vi "Command_Turn_To_Heading.vi"(0 "Startup":bool, 2 "Heading":dbl, 3 "Timeout":dbl=3.0) -> (5 "Reinit":bool, 6 "Completed":bool=TRUE, 7 "Speeds":dbl[](array[numeric]))   [LabVIEW 2018]
uses:
  Global_Variables/Sensor_Values.vi
panel:
  in  "Kd":dbl=0.0012 format="%#_13g"
  in  "Ki":dbl=0.0001 format="%#_13g"
  in  "Kp":dbl=0.01 format="%#_13g"
  out "Waveform Chart":cluster{"Heading":dbl, "Yaw":dbl}(graph)
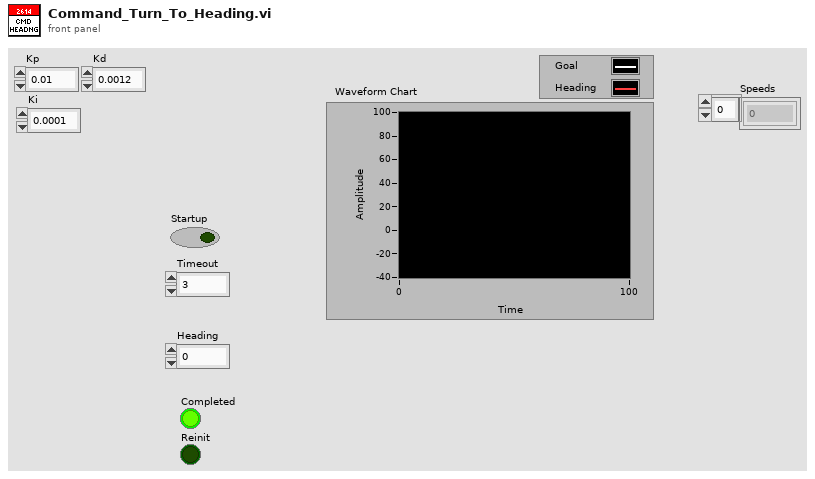
[diagram p1: front panel]
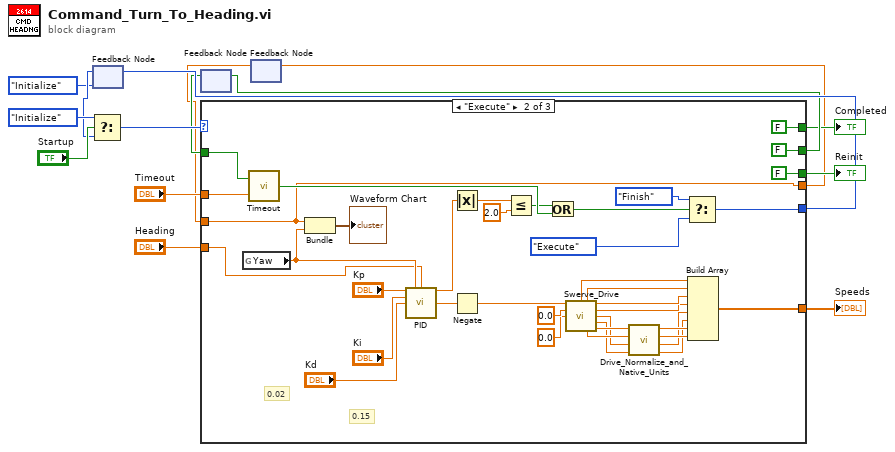
[diagram p0: block diagram]
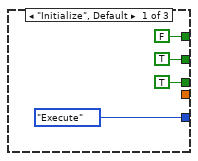
[diagram p2: hidden frame]
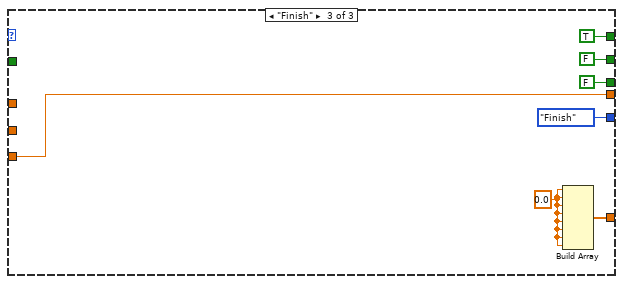
[diagram p3: hidden frame]
diagram:
  n1 = feedback #1(enum16{"Initialize", "Execute", "Finish"}."Initialize" ("f")) -> (w11:enum16{"Initialize", "Execute", "Finish"})
  n2 = Select(t=enum16{"Initialize", "Execute", "Finish"}."Initialize", s="Startup", f=w11) -> (s? t:f=w15:enum16{"Initialize", "Execute", "Finish"})
  n3 = feedback #2() -> (w9:bool)  [unwired: 1 in]
  n4 = feedback #3() -> (w1:dbl)  [unwired: 1 in]
  n5 = case shown="\"Execute\"" w15 {
    tunnel: [enum16{"Initialize", "Execute", "Finish"}."Execute" w54 enum16{"Initialize", "Execute", "Finish"}."Finish" ("f")] -> w12
    tunnel: w9 -> [_ w52 _]
    tunnel: [TRUE FALSE FALSE] -> w10
    tunnel: [FALSE FALSE TRUE] -> w8
    tunnel: [TRUE FALSE FALSE] -> w7
    tunnel: "Timeout" -> [_ w48 _]
    tunnel: "Heading" -> [_ w28 w58]
    tunnel: [_ w43 w60] -> w3
    tunnel: [_ w31 w58] -> w2
    tunnel: w1 -> [_ w31 _]
    frame "Initialize", Default {
    }
    frame "Execute" {
      # "0.02"
      # "0.15"
      n6 = global read "Sensor_Values.vi" "Yaw"() -> (w39:dbl)
      n7 = call "Timeout.vi"("Timeout"=w48, "Initialize"=w52) -> ("Timed Out?"=w49:bool)
      n8 = Bundle("Heading"=w31, "Yaw"=w39) -> (→"Waveform Chart":cluster{"Heading":dbl, "Yaw":dbl})  [unwired: 1 in]
      n9 = call "PID.vi"("Kp"="Kp", "Process Variable"=w39, "Goal"=w28, "Ki"="Ki", "Kd"="Kd") -> ("Current Error"=w30:dbl, "Command"=w33:dbl)  [unwired: 8 in, 1 out]
      n10 = Absolute Value(x=w30) -> (abs(x)=w29:dbl)
      n11 = Negate(x=w33) -> (-x=w32:dbl)
      n12 = Less Or Equal?(x=w29, y=2.0) -> (x <= y?=w37:bool)
      n13 = Or(x=w37, y=w49) -> (x .or. y?=w50:bool)
      n14 = call "Swerve_Drive.vi"("Z"=w32, "Y"=0.0, "X"=0.0) -> ("Back Left Spin Speed"=w47:dbl, "Back Right Spin Speed"=w46:dbl, "Front Left Spin Speed"=w45:dbl, "Front Right Spin Speed"=w44:dbl, "Back Left Motor Power"=w21:dbl, "Back Right Motor Power"=w23:dbl, "Front Right Motor Power"=w27:dbl, "Front Left Motor Power"=w25:dbl)  [unwired: 5 in]
      n15 = call "Drive_Normalize_and_Native_Units.vi"("BR"=w23, "BL"=w21, "FR"=w27, "FL"=w25) -> ("BR_Out"=w22:dbl, "BL_Out"=w20:dbl, "FR_Out"=w26:dbl, "FL_Out"=w24:dbl)
      n16 = Select(t=enum16{"Initialize", "Execute", "Finish"}."Finish", s=w50, f=enum16{"Initialize", "Execute", "Finish"}."Execute") -> (s? t:f=w54:enum16{"Initialize", "Execute", "Finish"})
      n17 = Build Array(w47, w46, w45, w44, w20, w22, w24, w26) -> (w43:dbl[])
    }
    frame "Finish" {
      w59 = 0.0 ("element")
      n18 = Build Array(w59, w59, w59, w59, w59, w59, w59, w59) -> (w60:dbl[])
    }
  }
  "Completed" <- w8
  "Reinit" <- w7
  "Speeds" <- w3
  n19 = feedback-in #1(w12) -> ()
  n20 = feedback-in #2(w10) -> ()
  n21 = feedback-in #3(w2) -> ()
